vi "Inflate DWT Coeff.vi"(8 "error in (no error)":errorcluster, 11 "data string":string) -> (0 "error out":errorcluster, 3 "Array":cluster{i32[][], i32[][], i32[][], i32[][]}[](array[cluster]))   [LabVIEW 2023]
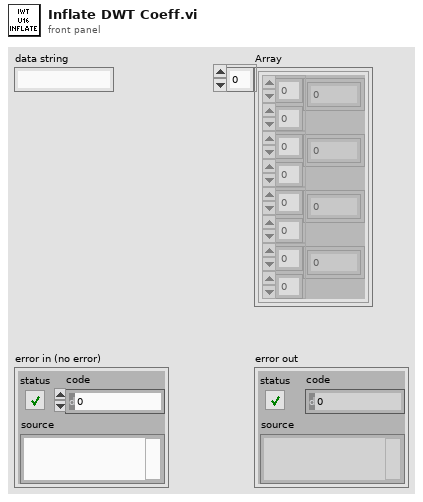
[diagram p1: front panel]
types:
  T1 = cluster{"[0]":cluster{i32[][]}, "[1]":cluster{i32[][]}, "[2]":cluster{i32[][]}, "[3]":cluster{i32[][]}}
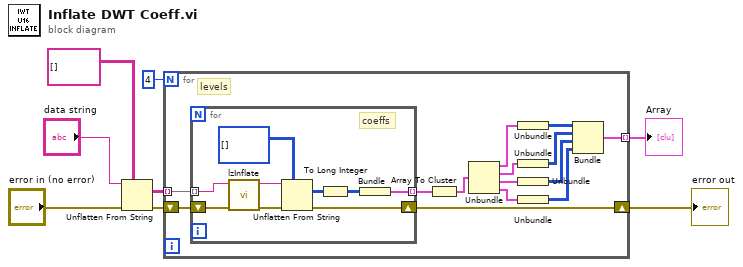
[diagram p0: block diagram]
diagram:
  n1 = Unflatten From String(type=string[][] [], binary string="data string", error in (no error)="error in (no error)") -> (value=w2:string[][], error out=w8:errorcluster)  [unwired: 2 in, 1 out]
  n2 = for {
    N: 4 -> [_]
    tunnel: w2 -> [w22] mode=indexing
    tunnel: [w11] -> w6 mode=indexing
    shift-right: [w9] -> w1
    shift-left: w8 -> [w10]
    # "levels"
    n3 = for {
      tunnel: w22 -> [w31] mode=indexing
      tunnel: [w28] -> w21 mode=indexing
      shift-right: [w23] -> w9
      shift-left: w10 -> [w25]
      # "coeffs"
      n4 = call "lzInflate.vi"("error in (no error)"=w25, "input"=w31) -> ("error out"=w24:errorcluster, "inflated output"=w30:string)  [unwired: 3 in, 1 out]
      n5 = Unflatten From String(type=i16[][] [], binary string=w30, error in (no error)=w24) -> (value=w27:i16[][], error out=w23:errorcluster)  [unwired: 2 in, 1 out]
      n6 = To Long Integer(number=w27) -> (32bit integer=w26:i32[][])
      n7 = Bundle(w26) -> (w28:cluster{i32[][]})  [unwired: 1 in]
    }
    n8 = Array To Cluster(array=w21) -> (cluster=w20:T1)
    n9 = Unbundle(w20) -> ("[0]"=w19:cluster{i32[][]}, "[1]"=w18:cluster{i32[][]}, "[2]"=w17:cluster{i32[][]}, "[3]"=w16:cluster{i32[][]})
    n10 = Unbundle(w19) -> (w15:i32[][])
    n11 = Unbundle(w18) -> (w14:i32[][])
    n12 = Unbundle(w17) -> (w13:i32[][])
    n13 = Unbundle(w16) -> (w12:i32[][])
    n14 = Bundle(w15, w14, w13, w12) -> (w11:cluster{i32[][], i32[][], i32[][], i32[][]})  [unwired: 1 in]
  }
  "error out" <- w1
  "Array" <- w6
